vi "Leap Open.vi"(8 "error in (no error)":errorcluster, 10 "Enable Gestures? (T)":bool=TRUE) -> (0 "error out":errorcluster, 3 "Leap Handle Out":T1)   [LabVIEW 2011, in "LVH-Leap.lvlib"]
doc: "Leap Open allows you to open a connection to the Leap Motion Controller with the option of having gestures enabled. When <b>Enable Gestures?</b> is true, all available gestures are turned on including Circle, Swipe, Screen Tap, and Key Tap detection.\n\nIf gestures are not being used then set <b>Enable Gestures?</b> to false to reduce the amount of resource utilization required by the Leap Motion for processing gestures."
uses:
  LVH-Leap.lvlib
  Private/Type Defs/Leap Handle.ctl
  C:/github/labviewhacker/LVH-Leap/LabVIEW/vi.lib/LabVIEW Hacker/Leap/Private/Libs/LeapCSharp.NET3.5.dll
  Private/Libs/LeapCSharp.NET3.5.dll
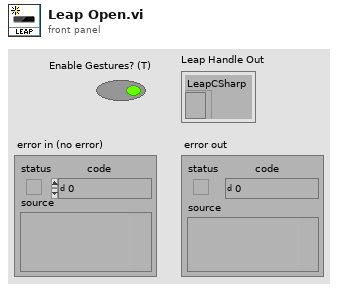
[diagram p1: front panel]
types:
  T1 = typedef "LVH-Leap.lvlib/Leap Handle.ctl" = cluster{"LeapCSharp":refnum<k24>}
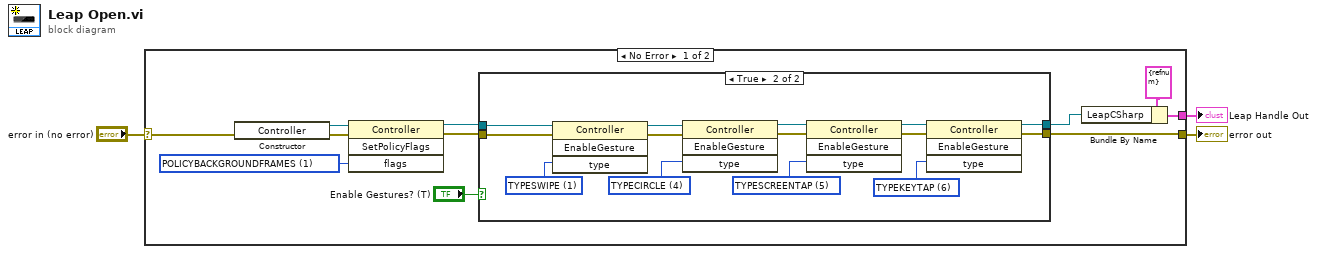
[diagram p0: block diagram]
diagram:
  n1 = case shown="No Error" "error in (no error)" {
    selector: "error in (no error)" -> [w14 w31]
    tunnel: [w11 w31] -> w2
    tunnel: [w12 _] -> w1
    frame No Error {
      w4 = 1 items=["POLICYDEFAULT", "POLICYBACKGROUNDFRAMES"] ("flags")
      n2 = constructor class="Controller"(error in=w14) -> (reference out=w5:refnum<k24>, error out=w8:errorcluster)  [unwired: 2 in, 1 out]
      n3 = invoke class="Controller" method="SetPolicyFlags"(reference=w5, error in=w8, "flags"=w4) -> (reference out=w6:refnum<k24>, error out=w7:errorcluster)  [unwired: 1 in, 2 out]
      n4 = case shown="True" "Enable Gestures? (T)" {
        tunnel: w6 -> [w15 w30]
        tunnel: w7 -> [w16 w29]
        tunnel: [w16 w28] -> w11
        tunnel: [w15 w27] -> w10
        frame False {
        }
        frame True {
          w19 = 6 items=["TYPESWIPE"=1, "TYPECIRCLE"=4, "TYPESCREENTAP"=5, "TYPEKEYTAP"=6, "TYPEINVALID"=-1] ("type")
          w22 = 5 items=["TYPESWIPE"=1, "TYPECIRCLE"=4, "TYPESCREENTAP"=5, "TYPEKEYTAP"=6, "TYPEINVALID"=-1] ("type")
          w23 = 4 items=["TYPESWIPE"=1, "TYPECIRCLE"=4, "TYPESCREENTAP"=5, "TYPEKEYTAP"=6, "TYPEINVALID"=-1] ("type")
          w26 = 1 items=["TYPESWIPE"=1, "TYPECIRCLE"=4, "TYPESCREENTAP"=5, "TYPEKEYTAP"=6, "TYPEINVALID"=-1] ("type")
          n5 = invoke class="Controller" method="EnableGesture"(reference=w30, error in=w29, "type"=w26) -> (reference out=w25:refnum<k24>, error out=w24:errorcluster)  [unwired: 1 in, 2 out]
          n6 = invoke class="Controller" method="EnableGesture"(reference=w25, error in=w24, "type"=w23) -> (reference out=w21:refnum<k24>, error out=w20:errorcluster)  [unwired: 1 in, 2 out]
          n7 = invoke class="Controller" method="EnableGesture"(reference=w21, error in=w20, "type"=w22) -> (reference out=w17:refnum<k24>, error out=w18:errorcluster)  [unwired: 1 in, 2 out]
          n8 = invoke class="Controller" method="EnableGesture"(reference=w17, error in=w18, "type"=w19) -> (reference out=w27:refnum<k24>, error out=w28:errorcluster)  [unwired: 1 in, 2 out]
        }
      }
      n9 = Bundle By Name(cluster=T1 {"LeapCSharp"=refnum} ("LeapController"), "LeapCSharp"=w10) -> (w12:T1)
    }
    frame Error {
    }
  }
  "error out" <- w2
  "Leap Handle Out" <- w1
